vi "Parse Model String.vi"(11 "read buffer":string) -> (2 "Found?":bool, 3 "token string":string)   [LabVIEW 2014]
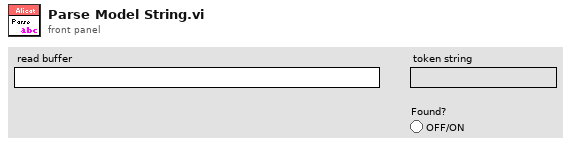
[diagram p1: front panel]
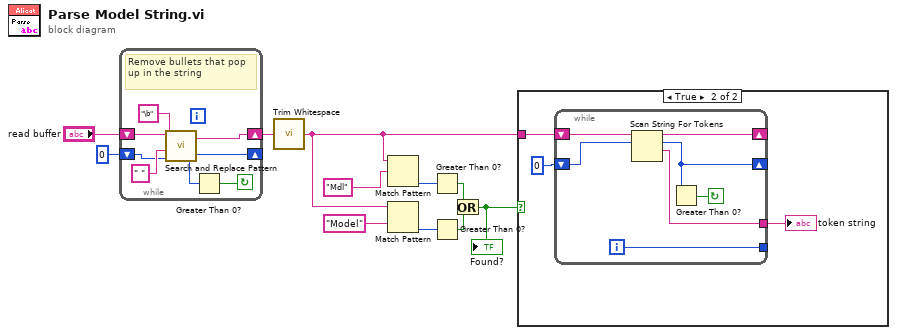
[diagram p0: block diagram]
diagram:
  n1 = while {
    shift-right: [w13] -> _
    shift-left: 0 ("offset past match") -> [w14]
    shift-right: [w15] -> w3
    shift-left: "read buffer" -> [w18]
    stop <- w12 continue-if-true
    # "Remove bullets that pop up in the string"
    n2 = call <vilib>:"Search and Replace Pattern.vi"("string"=w18, "regular expression (\"\")"="\b" ("regular expression (\"\")"), "replace string (\"\")"=" " ("replace string (\"\")"), "offset (0)"=w14) -> ("result string"=w15:string, "offset past match"=w13:i32)  [unwired: 1 in]
    n3 = Greater Than 0?(x=w13) -> (x > 0?=w12:bool)
  }
  n4 = call <vilib>:"Trim Whitespace.vi"("string"=w3) -> ("trimmed string"=w1:string)  [unwired: 1 in]
  n5 = Match Pattern(string=w1, regular expression="Mdl") -> (offset past match=w9:i32)  [unwired: 1 in, 3 out]
  n6 = Match Pattern(string=w1, regular expression="Model") -> (offset past match=w8:i32)  [unwired: 1 in, 3 out]
  n7 = Greater Than 0?(x=w9) -> (x > 0?=w7:bool)
  n8 = Greater Than 0?(x=w8) -> (x > 0?=w6:bool)
  n9 = Or(x=w7, y=w6) -> (x .or. y?=w5:bool)
  "Found?" <- w5
  n10 = case shown="True" w5 {
    tunnel: w1 -> [_ w21]
    frame False {
    }
    frame True {
      n11 = while {
        shift-right: [w26] -> _
        shift-left: w21 -> [w27]
        shift-right: [w25] -> _
        shift-left: 0 ("offset past token") -> [w24]
        tunnel: [w23] -> w19
        tunnel: [w22] -> _
        i -> [w22]
        stop <- w28 continue-if-true
        n12 = Scan String For Tokens(8:w24, 9:w27) -> (1:w23:string, 2:w25:i32, 3:w26:string)  [unwired: 4 in, 1 out]
        n13 = Greater Than 0?(x=w25) -> (x > 0?=w28:bool)
      }
      "token string" <- w19
    }
  }
